vi "Filter Tree.vi"(7 "Headers":string[](array[string]), 8 "error in":errorcluster, 9 "Tags map":refnum<vi>, 10 "Frames":refnum<vi>, 11 "Filter":refnum<vi>) -> (0 "error out":errorcluster)   [LabVIEW 2025, in "CAN-LIN Raw Bus Capture UI.lvlib"]
uses:
  CAN-LIN Raw Bus Capture UI.lvlib
  <vilib>/Utility/error.llb/whitespace.ctl
  <vilib>/Utility/error.llb/Trim Whitespace One-Sided.vi
  Table_Filtering/Table_Filtering.lvlib
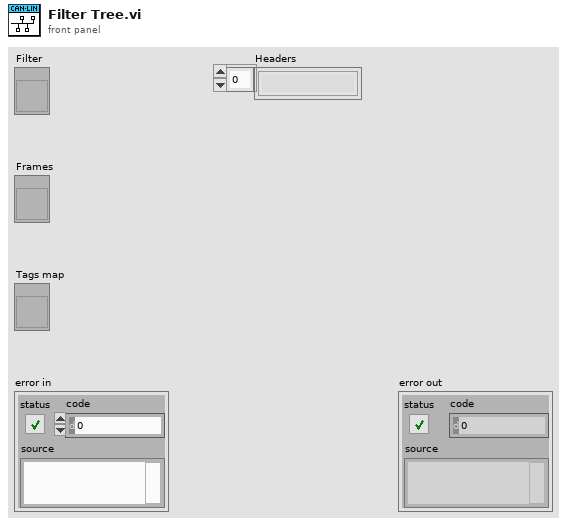
[diagram p1: front panel]
types:
  T1 = typedef "whitespace.ctl" = u16
  T2 = cluster{"FIELD":string, "OPERATOR":string, "VALUE":string}[]
  T3 = cluster{"Array":string[], "appended array":string[][]}[]
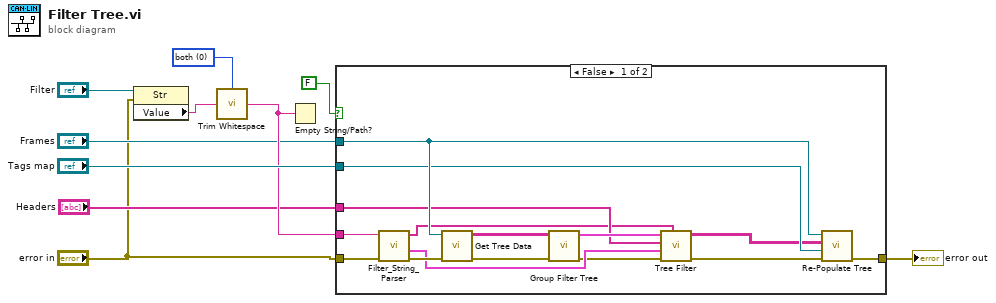
[diagram p0: block diagram]
diagram:
  w6 = T1 0 items=["both", "start of string", "end of string"] ("location (both)")
  n1 = property class="Str"(reference="Filter", error in="error in") -> ("Value"=w10:string)  [unwired: 2 out]
  n2 = call <vilib>:"Trim Whitespace.vi"("string"=w10, "location (both)"=w6) -> ("trimmed string"=w7:string)
  n3 = Empty String/Path?(string/path=w7) -> ()  [unwired: 1 out]
  n4 = case shown="False" FALSE {
    tunnel: "error in" -> [w25 w26]
    tunnel: "Headers" -> [w17 _]
    tunnel: "Frames" -> [w23 _]
    tunnel: [w22 w26] -> w5
    tunnel: w7 -> [w21 _]
    tunnel: "Tags map" -> [w20 _]
    frame False {
      n5 = call "Filter_String_Parser.vi"("error in"=w25, "Filter String"=w21) -> ("error constant"=w24:errorcluster, "Comparators"=w16:T2, "Boolean Connectors"=w15:string[])  [unwired: 7 in]
      n6 = call "Get Tree Data.vi"("error in"=w24, "Tree ref"=w23) -> ("error out"=w12:errorcluster, "Array"=w19:string[][])  [unwired: 8 in]
      n7 = call "Group Filter Tree.vi"("error in"=w12, "Data in"=w19) -> ("error IO"=w11:errorcluster, "Frame groups"=w18:T3)  [unwired: 8 in]
      n8 = call "Tree Filter.vi"("Boolean Connectors"=w15, "error in"=w11, "Comparators"=w16, "Headers"=w17, "Frame groups"=w18) -> ("error out"=w14:errorcluster, "Filtered tree"=w13:string[][])  [unwired: 5 in]
      n9 = call "Re-Populate Tree.vi"("error in"=w14, "Tags map"=w20, "Data in"=w13, "TreeControl in"=w23) -> ("error out"=w22:errorcluster)  [unwired: 7 in]
    }
    frame True {
    }
  }
  "error out" <- w5
